vi "TranslatorBooster Is String Datatype.vi"(1 "String token":string) -> (0 "Is datatype?":bool)   [LabVIEW 2014, in "Complex Numbers.lvlib"]
uses:
  <vilib>/Aledyne-TSXperts/Arduino Compatible Compiler for LabVIEW/addons/Complex Numbers/Complex Numbers.lvlib
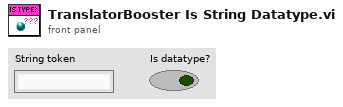
[diagram p1: front panel]
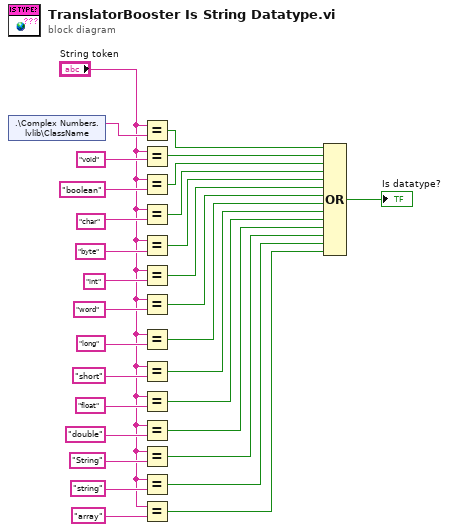
[diagram p0: block diagram]
diagram:
  n1 = shared-variable ".\\Complex Numbers.lvlib\\ClassName"() -> (w22:string)  [unwired: 1 in, 1 out]
  n2 = Equal?(x="String token", y=w22) -> (x = y?=w26:bool)
  n3 = Equal?(x="String token", y="void") -> (x = y?=w27:bool)
  n4 = Equal?(x="String token", y="boolean") -> (x = y?=w28:bool)
  n5 = Equal?(x="String token", y="char") -> (x = y?=w29:bool)
  n6 = Equal?(x="String token", y="byte") -> (x = y?=w10:bool)
  n7 = Equal?(x="String token", y="int") -> (x = y?=w9:bool)
  n8 = Equal?(x="String token", y="word") -> (x = y?=w8:bool)
  n9 = Equal?(x="String token", y="long") -> (x = y?=w7:bool)
  n10 = Equal?(x="String token", y="short") -> (x = y?=w6:bool)
  n11 = Equal?(x="String token", y="float") -> (x = y?=w5:bool)
  n12 = Equal?(x="String token", y="double") -> (x = y?=w4:bool)
  n13 = Equal?(x="String token", y="String") -> (x = y?=w3:bool)
  n14 = Equal?(x="String token", y="string") -> (x = y?=w2:bool)
  n15 = Equal?(x="String token", y="array") -> (x = y?=w1:bool)
  n16 = Compound Arithmetic op=OR(w26, w27, w28, w29, w10, w9, w8, w7, w6, w5, w4, w3, w2, w1) -> (→"Is datatype?":bool)
